vi "Fetch Read Buffer Statistics.vi"(0 "VISA resource name":refnum<visa-resource-name>, 5 "Buffer Name (defbuffer1)":string="defbuffer1", 7 "Statistical Operation (0: Mean)":u16(ring) items=["Mean", "Standard Deviation", "Maximum", "Minimum", "Peak to Peak"], 11 "error in (no error)":errorcluster) -> (4 "VISA resource name out":refnum<visa-resource-name>, 6 "Data Out":dbl, 15 "error out":errorcluster)   [LabVIEW 2020, in "Keithley 2450.lvlib"]
doc: "This gives the statistical information associated with the specified buffer."
uses:
  <instrlib>/Keithley 2450/Keithley 2450.lvlib
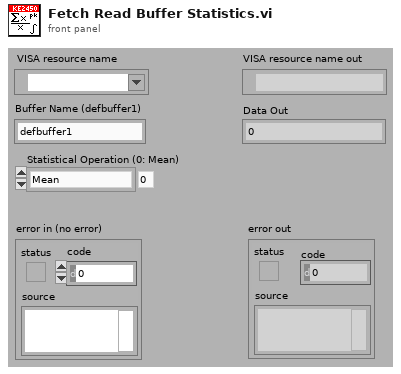
[diagram p1: front panel]
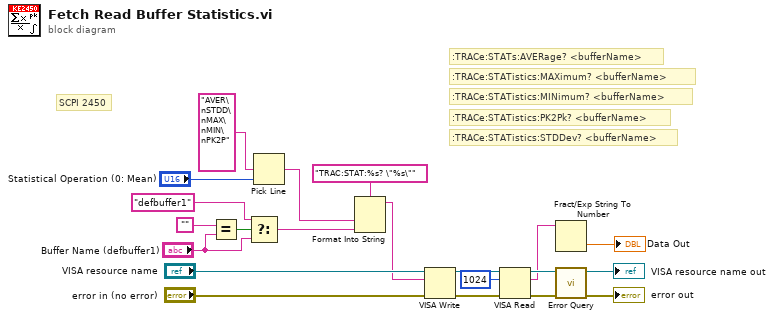
[diagram p0: block diagram]
diagram:
  # ":TRACe:STATistics:STDDev? <bufferName>"
  # ":TRACe:STATistics:PK2Pk? <bufferName>"
  # ":TRACe:STATistics:MINimum? <bufferName>"
  # ":TRACe:STATistics:MAXimum? <bufferName>"
  # ":TRACe:STATs:AVERage? <bufferName>"
  # "SCPI 2450"
  n1 = Equal?(x="", y="Buffer Name (defbuffer1)") -> (x = y?=w19:bool)
  n2 = Select(t="defbuffer1", s=w19, f="Buffer Name (defbuffer1)") -> (s? t:f=w16:string)
  n3 = Pick Line(multi-line string="AVER\nSTDD\nMAX\nMIN\nPK2P" ("t"), line index="Statistical Operation (0: Mean)") -> (output string=w8:string)  [unwired: 1 in]
  n4 = Format Into String(format string="TRAC:STAT:%s? \"%s\"" ("Read Measurement"), w8, w16) -> (resulting string=w11:string)  [unwired: 2 in, 1 out]
  n5 = VISA Write(VISA resource name="VISA resource name", write buffer=w11, error in (no error)="error in (no error)") -> (VISA resource name out=w5:refnum<visa-resource-name>, error out=w7:errorcluster)  [unwired: 1 out]
  n6 = VISA Read(VISA resource name=w5, byte count=u32 1024, error in (no error)=w7) -> (VISA resource name out=w4:refnum<visa-resource-name>, read buffer=w2:string, error out=w6:errorcluster)  [unwired: 1 out]
  n7 = Fract/Exp String To Number(string=w2) -> (number=→"Data Out":dbl)  [unwired: 3 in, 1 out]
  n8 = call <instrlib>:"Error Query.vi"("error in (no error)"=w6, "VISA resource name"=w4) -> ("error out"=→"error out":errorcluster, "VISA resource name out"=→"VISA resource name out":refnum<visa-resource-name>)  [unwired: 8 out]
